vi "Score L3.vi"(9 "Combo Box":string(combo)) -> (0 "Done":bool)   [LabVIEW 2020]
uses:
  <vilib>/Rock Robotics/WPI/Utilities/WPI_GetSetVariantRefNum.vi
  Robot Global Data.vi
  <vilib>/Rock Robotics/WPI/RobotDrive/WPI_RobotDriveArcadeDrive_Standard(NoSaturation).vi
panel:
  out "Done":bool
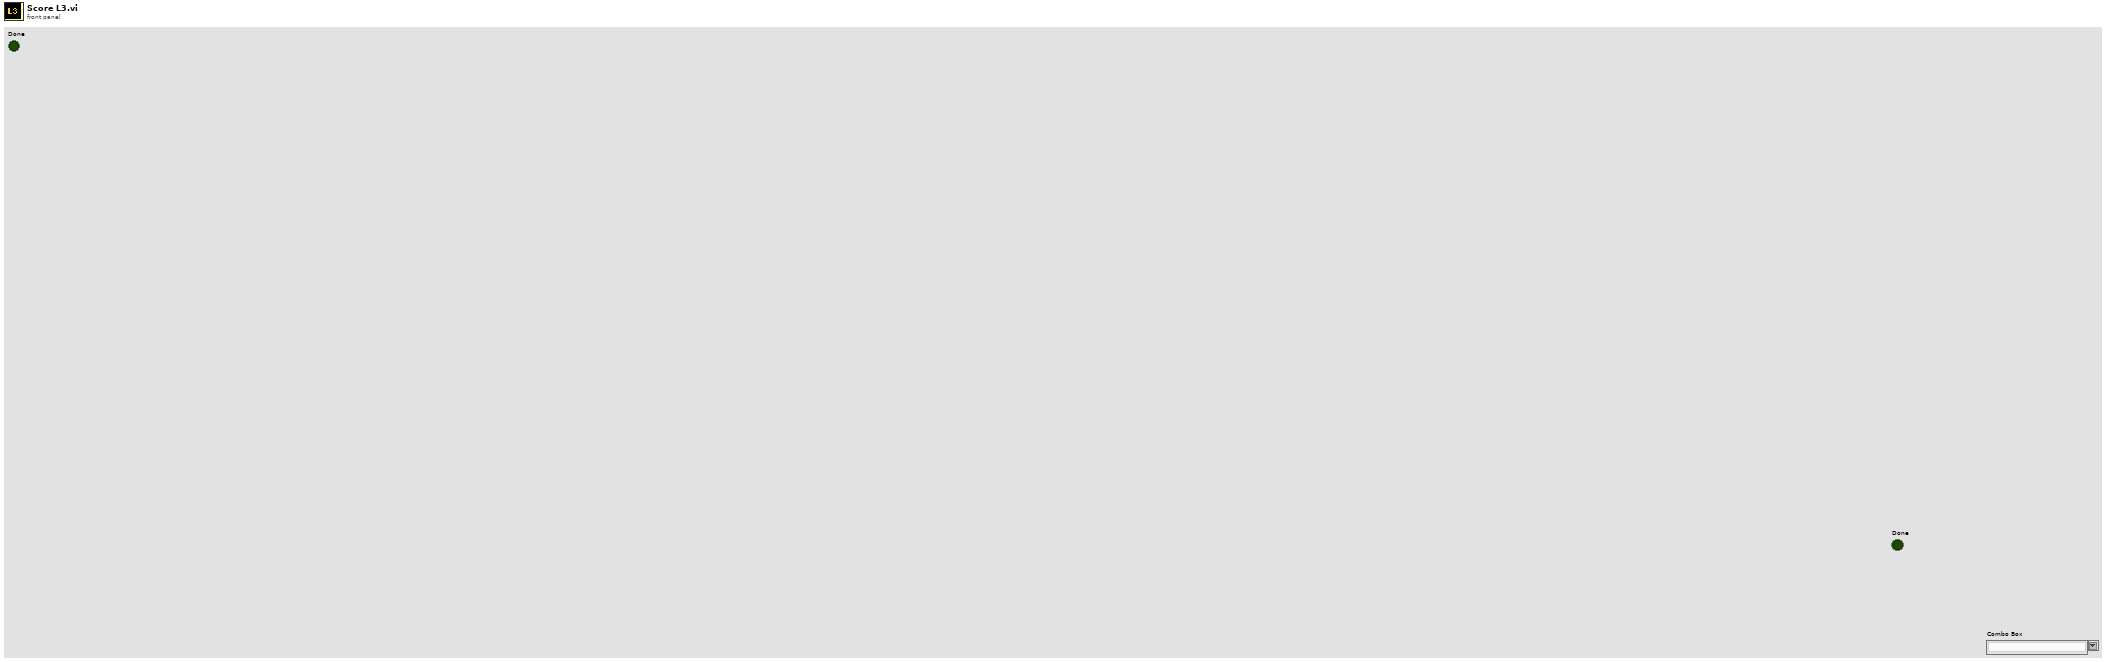
[diagram p1: front panel]
types:
  T1 = typedef "WPI_MotorControlDeviceRef.ctl" = cluster{"DeviceStatus":errorcluster, "Type":T2, "PWM":cluster{"PWM Channel":T3, "DeadBand":T4}, "CAN":cluster{"Device Number":u8, "SetOutput VI Ref":variant, "GetOutput VI Ref":variant, "Enable VI Ref":variant, "Disable VI Ref":variant, "Data":variant}, "Invert":bool, "DIO PWM":cluster{"PWM \"Enable\" Channel":T3, "DIOChannel":T5, "PWM Rate":dbl}}
  T2 = typedef "WPI_MotorControlType.ctl" = enum16{"PWM", "CAN", "DIO PWM"}
  T3 = typedef "FPGA_DIOPWMChannel.ctl" = enum8{"PWM 0", "PWM 1", "PWM 2", "PWM 3", "PWM 4", "PWM 5", "PWM 6", "PWM 7", "PWM 8", "PWM 9", "PWM MXP 0", "PWM MXP 1", "PWM MXP 2", "PWM MXP 3", "PWM MXP 4", "PWM MXP 5", "PWM MXP 6", "PWM MXP 7", "PWM MXP 8", "PWM MXP 9", "Invalid"}
  T4 = typedef "WPI_PWMDeadband.ctl" = cluster{"Name":string, "maxPositivePwm":i32, "minPositivePwm":i32, "centerPwm":i32, "maxNegativePwm":i32, "minNegativePwm":i32, "angularRange":u16}
  T5 = typedef "FPGA_DIOChannel.ctl" = enum8{"DIO 0", "DIO 1", "DIO 2", "DIO 3", "DIO 4", "DIO 5", "DIO 6", "DIO 7", "DIO 8", "DIO 9", "DIO MXP 0", "DIO MXP 1", "DIO MXP 2", "DIO MXP 3", "DIO MXP 4", "DIO MXP 5", "DIO MXP 6", "DIO MXP 7", "DIO MXP 8", "DIO MXP 9", "DIO MXP 10", "DIO MXP 11", "DIO MXP 12", "DIO MXP 13", "DIO MXP 14", "DIO MXP 15", "SPI Port CS1", "SPI Port CS2", "SPI Port CS3", "SPI Port MISO", "SPI Port MOSI", "Invalid"}
  T6 = typedef "ADIS16470 Device Reference.ctl" = cluster{"DevStatus":errorcluster, "Hardware Config":T7, "Calibration Complete":refnum<notifier>, "Status Reference":refnum<data-value>, "Data Reference":refnum<data-value>, "Sychronous Process VI":T10, "Cmd FIFO":refnum<k33>, "Source":T11, "Data FIFO":refnum<k33>, "Calibration Time (ms)":u32, "Data Reference":refnum<data-value>}
  T7 = typedef "ADIS16470 Hardware Configuration.ctl" = cluster{"SPI Clock Rate (Hz)":dbl, "IMU SPI Mode (3)":T8, "IMU Reset Pin":T5, "IMU SPI Bus":T9, "IMU Data Ready Pin":T5, "Stall Config":cluster{"Pow2BytesPerRead":u8, "StallTicks":u16, "CsToSclkTicks":u8}}
  T8 = typedef "WPI_SPIMode.ctl" = enum16{"Mode 0 (Clk Idle Low,Sample on Leading)", "Mode 1 (Clk Idle Low,Sample on Trailing)", "Mode 2 (Clk Idle High,Sample on Leading)", "Mode 3 (Clk Idle High,Sample on Trailing)"}
  T9 = typedef "spi_bus.ctl" = enum16{"SPI On-Board, CS0", "SPI On-Board, CS1", "SPI On-Board, CS2", "SPI On-Board, CS3", "SPI MXP", "Invalid"}
  T10 = typedef "ADIS16470 Process.ctl" = refnum<vi>
  T11 = typedef "FPGA_CounterEncoderSourceConvertionLVSourceType.ctl" = cluster{"DevStatus":errorcluster, "AnalogTriggerMode?":bool, "DigitalMode":cluster{"DIO Channel":T12}, "AnalogTriggerMode":cluster{"AnalogTriggerIndex":T13, "OutputType":T14}}
  T12 = typedef "FPGA_DIODigitalSourceChannel.ctl" = enum8{"DIO 0", "DIO 1", "DIO 2", "DIO 3", "DIO 4", "DIO 5", "DIO 6", "DIO 7", "DIO 8", "DIO 9", "DIO MXP 0", "DIO MXP 1", "DIO MXP 2", "DIO MXP 3", "DIO MXP 4", "DIO MXP 5", "DIO MXP 6", "DIO MXP 7", "DIO MXP 8", "DIO MXP 9", "DIO MXP 10", "DIO MXP 11", "DIO MXP 12", "DIO MXP 13", "DIO MXP 14", "DIO MXP 15", "SPI Port CS1", "SPI Port CS2", "SPI Port CS3", "SPI Port MISO", "SPI Port MOSI", "Disabled"}
  T13 = typedef "FPGA_AnalogTriggerIndex.ctl" = enum8{"Trig 0", "Trig 1", "Trig 2", "Trig 3", "Trig 4", "Trig 5", "Trig 6", "Trig 7", "Invalid"}
  T14 = typedef "FPGA_AnalogTriggerOutType.ctl" = enum16{"InWindow", "TriggerState", "Rising", "Falling"}
  T15 = typedef "WPI_RobotDriveDevRef.ctl" = cluster{"DevStatus":errorcluster, "Motors[]":T1[], "Square Inputs":bool, "Max Output":dbl}
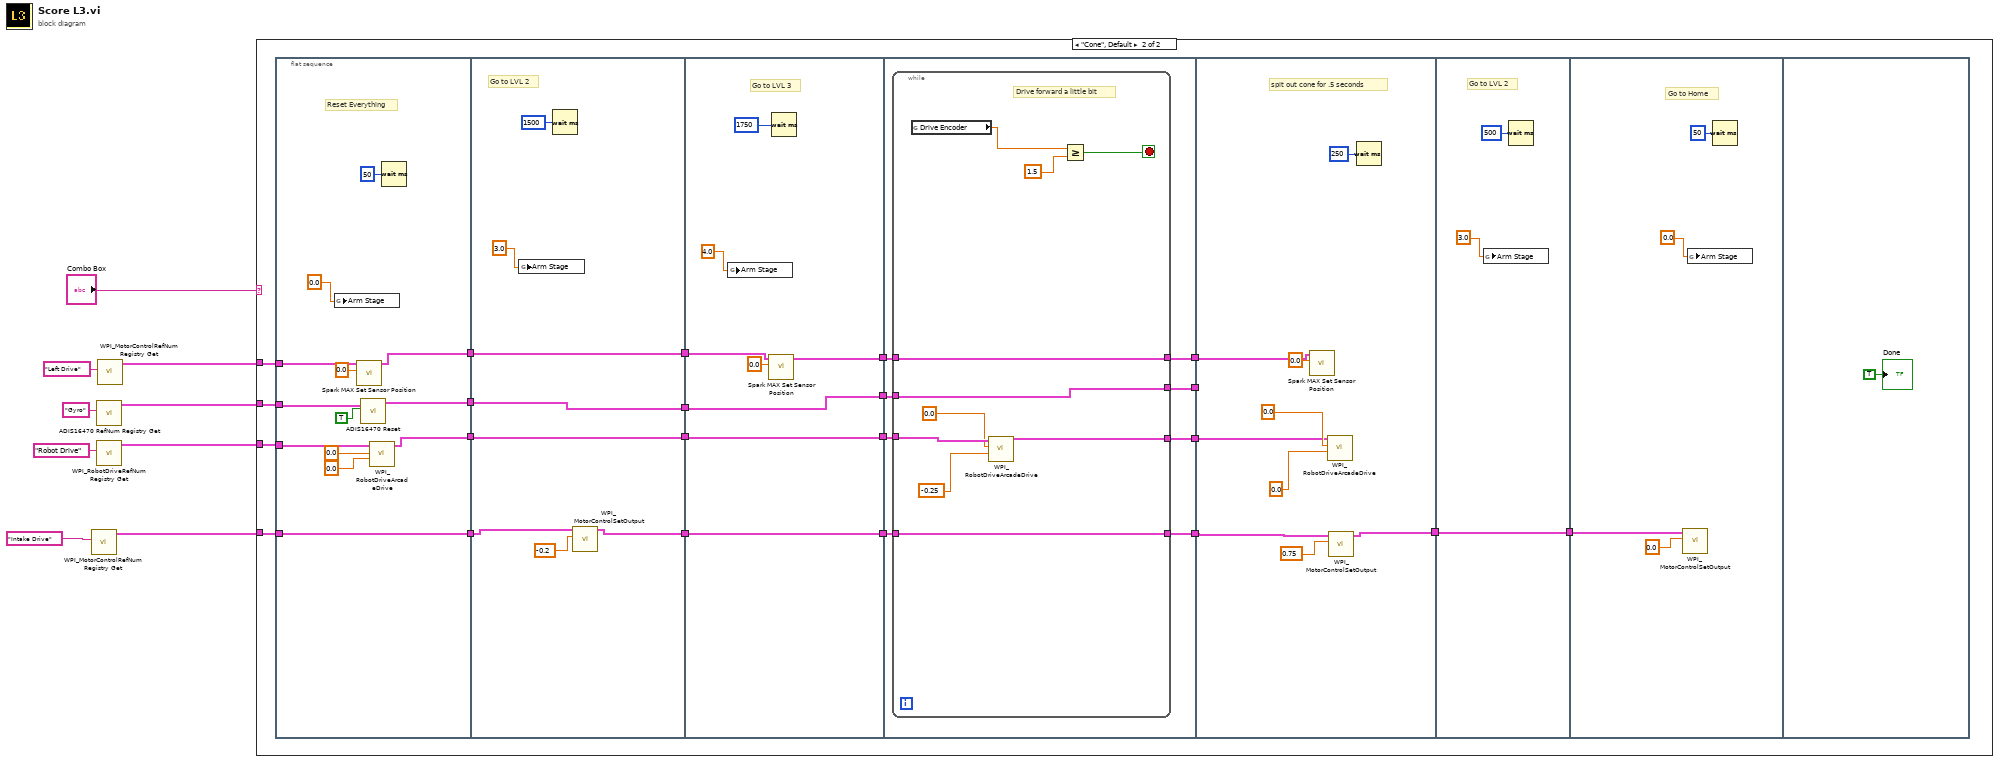
[diagram p0: block diagram]
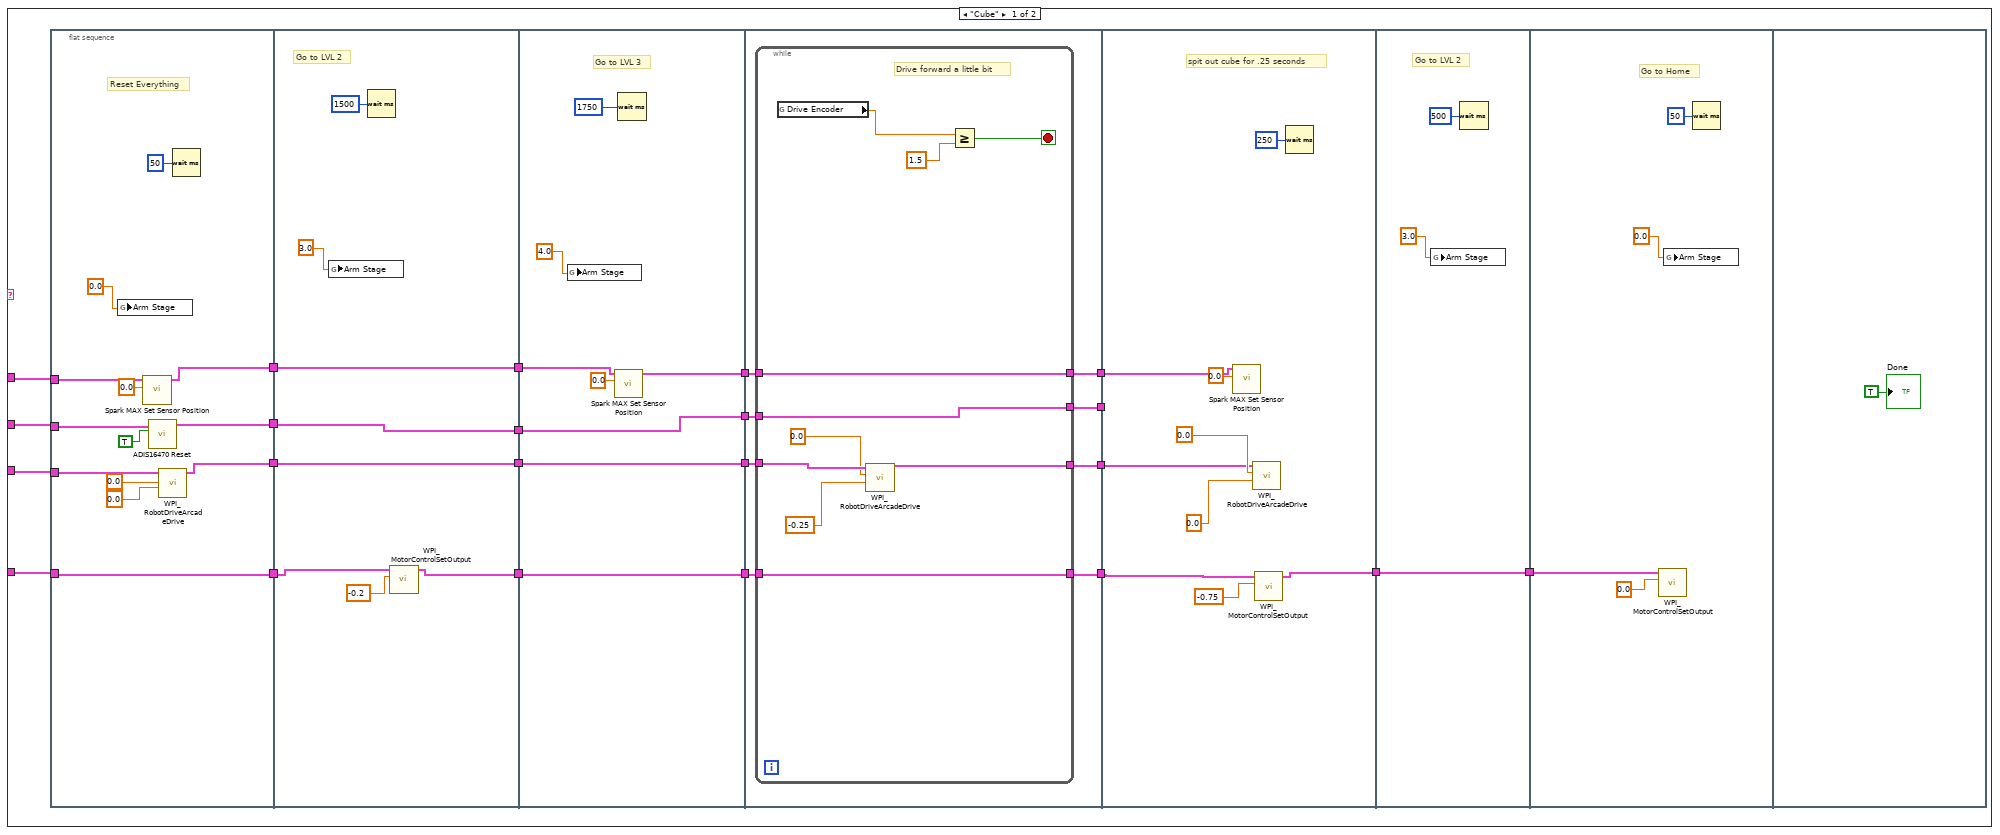
[diagram p2: hidden frame]
diagram:
  n1 = call <vilib>:"WPI_MotorControlRefNum Registry Get.vi"("refnum name"="Intake Drive") -> ("MotorControlDevRef"=w2:T1)  [unwired: 9 in, 1 out]
  n2 = call <vilib>:"ADIS16470 RefNum Registry Get.vi"("refnum name"="Gyro") -> ("ADIS16470DevRef out"=w4:T6)  [unwired: 9 in, 1 out]
  n3 = call <vilib>:"WPI_RobotDriveRefNum Registry Get.vi"("refnum name"="Robot Drive") -> ("RobotDriveDevRef"=w3:T15)  [unwired: 9 in, 1 out]
  n4 = call <vilib>:"WPI_MotorControlRefNum Registry Get.vi"("refnum name"="Left Drive") -> ("MotorControlDevRef"=w5:T1)  [unwired: 9 in, 1 out]
  n5 = case shown="\"Cone\", Default" "Combo Box" {
    tunnel: w5 -> [w13 w99]
    tunnel: w4 -> [w12 w98]
    tunnel: w3 -> [w11 w97]
    tunnel: w2 -> [w10 w96]
    frame "Cube" {
      n6 = flat-sequence {
        tunnel: w11 -> [w44]
        tunnel: w13 -> [w41]
        tunnel: w12 -> [w39]
        tunnel: [w35] -> w31
        tunnel: [w34] -> w30
        tunnel: w10 -> [w34]
        tunnel: [w33] -> w29
        tunnel: [w32] -> w28
        tunnel: [w50] -> w27
        tunnel: w31 -> [w50]
        tunnel: w30 -> [w46]
        tunnel: [w45] -> w26
        tunnel: [w49] -> w25
        tunnel: w29 -> [w49]
        tunnel: [w48] -> w24
        tunnel: w28 -> [w48]
        tunnel: [w58] -> w23
        tunnel: w27 -> [w58]
        tunnel: [w53] -> w22
        tunnel: w26 -> [w53]
        tunnel: w25 -> [w56]
        tunnel: [w55] -> w21
        tunnel: [w54] -> w20
        tunnel: w24 -> [w54]
        tunnel: w23 -> [w68]
        tunnel: w22 -> [w67]
        tunnel: [w66] -> w19
        tunnel: [w65] -> w18
        tunnel: [w64] -> w17
        tunnel: w21 -> [w63]
        tunnel: [w62] -> w16
        tunnel: w20 -> [w61]
        tunnel: w19 -> [w84]
        tunnel: w18 -> [w83]
        tunnel: w17 -> [w80]
        tunnel: w16 -> [_]
        tunnel: [w79] -> w15
        tunnel: [w88] -> w14
        tunnel: w15 -> [w88]
        tunnel: w14 -> [w92]
        frame #0 {
          # "Reset Everything"
          n7 = global write "Robot Global Data.vi" "Arm Stage"(0.0 ("Arm Stage")) -> ()
          n8 = call <vilib>:"Spark MAX Set Sensor Position.vi"("Position"=0.0, "MotorControlDeviceRef"=w41) -> ("MotorControlDeviceRef"=w33:T1)  [unwired: 8 in, 1 out]
          n9 = call <vilib>:"ADIS16470 Reset.vi"("Reset? (T)"=TRUE, "ADIS16470DevRef"=w39) -> ("ADIS16470DevRef"=w32:T6)  [unwired: 8 in, 1 out]
          n10 = call-poly <vilib>:"WPI_RobotDriveArcadeDrive.vi"("Y axis value"=0.0, "X axis value"=0.0, "RobotDriveDevRef"=w44) -> ("RobotDriveDevRef"=w35:T15)  [unwired: 6 in, 2 out]
          n11 = Wait (ms)(milliseconds to wait=u32 50) -> ()  [unwired: 1 out]
        }
        frame #1 {
          # "Go to LVL 2"
          n12 = global write "Robot Global Data.vi" "Arm Stage"(3.0 ("Arm Stage")) -> ()
          n13 = Wait (ms)(milliseconds to wait=u32 1500) -> ()  [unwired: 1 out]
          n14 = call <vilib>:"WPI_MotorControlSetOutput.vi"("Output"=-0.2, "MotorControlDevRef"=w46) -> ("MotorControlDevRef"=w45:T1)  [unwired: 7 in, 2 out]
        }
        frame #2 {
          # "Go to LVL 3"
          n15 = global write "Robot Global Data.vi" "Arm Stage"(4.0 ("Arm Stage")) -> ()
          n16 = call <vilib>:"Spark MAX Set Sensor Position.vi"("Position"=0.0, "MotorControlDeviceRef"=w56) -> ("MotorControlDeviceRef"=w55:T1)  [unwired: 8 in, 1 out]
          n17 = Wait (ms)(milliseconds to wait=u32 1750) -> ()  [unwired: 1 out]
        }
        frame #3 {
          n18 = while {
            tunnel: w68 -> [w78]
            tunnel: w67 -> [w72]
            tunnel: [w72] -> w66
            tunnel: [w71] -> w65
            tunnel: [w70] -> w64
            tunnel: w63 -> [w70]
            tunnel: [w69] -> w62
            tunnel: w61 -> [w69]
            stop <- w73 stop-if-true
            # "Drive forward a little bit"
            n19 = global read "Robot Global Data.vi" "Drive Encoder"() -> (w75:dbl)
            n20 = call-poly <vilib>:"WPI_RobotDriveArcadeDrive.vi"("Y axis value"=-0.25, "X axis value"=0.0, "RobotDriveDevRef"=w78) -> ("RobotDriveDevRef"=w71:T15)  [unwired: 6 in, 2 out]
            n21 = Greater Or Equal?(x=w75, y=1.5) -> (x >= y?=w73:bool)
          }
        }
        frame #4 {
          # "spit out cube for .25 seconds"
          n22 = call <vilib>:"Spark MAX Set Sensor Position.vi"("Position"=0.0, "MotorControlDeviceRef"=w80) -> ()  [unwired: 8 in, 2 out]
          n23 = call-poly <vilib>:"WPI_RobotDriveArcadeDrive.vi"("Y axis value"=0.0, "X axis value"=0.0, "RobotDriveDevRef"=w83) -> ()  [unwired: 6 in, 3 out]
          n24 = call <vilib>:"WPI_MotorControlSetOutput.vi"("Output"=-0.75, "MotorControlDevRef"=w84) -> ("MotorControlDevRef"=w79:T1)  [unwired: 7 in, 2 out]
          n25 = Wait (ms)(milliseconds to wait=u32 250) -> ()  [unwired: 1 out]
        }
        frame #5 {
          # "Go to LVL 2"
          n26 = global write "Robot Global Data.vi" "Arm Stage"(3.0 ("Arm Stage")) -> ()
          n27 = Wait (ms)(milliseconds to wait=u32 500) -> ()  [unwired: 1 out]
        }
        frame #6 {
          # "Go to Home"
          n28 = call <vilib>:"WPI_MotorControlSetOutput.vi"("Output"=0.0, "MotorControlDevRef"=w92) -> ()  [unwired: 7 in, 3 out]
          n29 = global write "Robot Global Data.vi" "Arm Stage"(0.0 ("Arm Stage")) -> ()
          n30 = Wait (ms)(milliseconds to wait=u32 50) -> ()  [unwired: 1 out]
        }
        frame #7 {
          "Done" <- TRUE ("Done")
        }
      }
    }
    frame "Cone", Default {
      n31 = flat-sequence {
        tunnel: w97 -> [w130]
        tunnel: w99 -> [w127]
        tunnel: w98 -> [w125]
        tunnel: [w121] -> w117
        tunnel: [w120] -> w116
        tunnel: w96 -> [w120]
        tunnel: [w119] -> w115
        tunnel: [w118] -> w114
        tunnel: [w136] -> w113
        tunnel: w117 -> [w136]
        tunnel: w116 -> [w132]
        tunnel: [w131] -> w112
        tunnel: [w135] -> w111
        tunnel: w115 -> [w135]
        tunnel: [w134] -> w110
        tunnel: w114 -> [w134]
        tunnel: [w144] -> w109
        tunnel: w113 -> [w144]
        tunnel: [w139] -> w108
        tunnel: w112 -> [w139]
        tunnel: w111 -> [w142]
        tunnel: [w141] -> w107
        tunnel: [w140] -> w106
        tunnel: w110 -> [w140]
        tunnel: w109 -> [w154]
        tunnel: w108 -> [w153]
        tunnel: [w152] -> w105
        tunnel: [w151] -> w104
        tunnel: [w150] -> w103
        tunnel: w107 -> [w149]
        tunnel: [w148] -> w102
        tunnel: w106 -> [w147]
        tunnel: w105 -> [w170]
        tunnel: w104 -> [w169]
        tunnel: w103 -> [w166]
        tunnel: w102 -> [_]
        tunnel: [w165] -> w101
        tunnel: [w174] -> w100
        tunnel: w101 -> [w174]
        tunnel: w100 -> [w178]
        frame #0 {
          # "Reset Everything"
          n32 = global write "Robot Global Data.vi" "Arm Stage"(0.0 ("Arm Stage")) -> ()
          n33 = call <vilib>:"Spark MAX Set Sensor Position.vi"("Position"=0.0, "MotorControlDeviceRef"=w127) -> ("MotorControlDeviceRef"=w119:T1)  [unwired: 8 in, 1 out]
          n34 = call <vilib>:"ADIS16470 Reset.vi"("Reset? (T)"=TRUE, "ADIS16470DevRef"=w125) -> ("ADIS16470DevRef"=w118:T6)  [unwired: 8 in, 1 out]
          n35 = call-poly <vilib>:"WPI_RobotDriveArcadeDrive.vi"("Y axis value"=0.0, "X axis value"=0.0, "RobotDriveDevRef"=w130) -> ("RobotDriveDevRef"=w121:T15)  [unwired: 6 in, 2 out]
          n36 = Wait (ms)(milliseconds to wait=u32 50) -> ()  [unwired: 1 out]
        }
        frame #1 {
          # "Go to LVL 2"
          n37 = global write "Robot Global Data.vi" "Arm Stage"(3.0 ("Arm Stage")) -> ()
          n38 = Wait (ms)(milliseconds to wait=u32 1500) -> ()  [unwired: 1 out]
          n39 = call <vilib>:"WPI_MotorControlSetOutput.vi"("Output"=-0.2, "MotorControlDevRef"=w132) -> ("MotorControlDevRef"=w131:T1)  [unwired: 7 in, 2 out]
        }
        frame #2 {
          # "Go to LVL 3"
          n40 = global write "Robot Global Data.vi" "Arm Stage"(4.0 ("Arm Stage")) -> ()
          n41 = call <vilib>:"Spark MAX Set Sensor Position.vi"("Position"=0.0, "MotorControlDeviceRef"=w142) -> ("MotorControlDeviceRef"=w141:T1)  [unwired: 8 in, 1 out]
          n42 = Wait (ms)(milliseconds to wait=u32 1750) -> ()  [unwired: 1 out]
        }
        frame #3 {
          n43 = while {
            tunnel: w154 -> [w164]
            tunnel: w153 -> [w158]
            tunnel: [w158] -> w152
            tunnel: [w157] -> w151
            tunnel: [w156] -> w150
            tunnel: w149 -> [w156]
            tunnel: [w155] -> w148
            tunnel: w147 -> [w155]
            stop <- w159 stop-if-true
            # "Drive forward a little bit"
            n44 = global read "Robot Global Data.vi" "Drive Encoder"() -> (w161:dbl)
            n45 = call-poly <vilib>:"WPI_RobotDriveArcadeDrive.vi"("Y axis value"=-0.25, "X axis value"=0.0, "RobotDriveDevRef"=w164) -> ("RobotDriveDevRef"=w157:T15)  [unwired: 6 in, 2 out]
            n46 = Greater Or Equal?(x=w161, y=1.5) -> (x >= y?=w159:bool)
          }
        }
        frame #4 {
          # "spit out cone for .5 seconds"
          n47 = call <vilib>:"Spark MAX Set Sensor Position.vi"("Position"=0.0, "MotorControlDeviceRef"=w166) -> ()  [unwired: 8 in, 2 out]
          n48 = call-poly <vilib>:"WPI_RobotDriveArcadeDrive.vi"("Y axis value"=0.0, "X axis value"=0.0, "RobotDriveDevRef"=w169) -> ()  [unwired: 6 in, 3 out]
          n49 = call <vilib>:"WPI_MotorControlSetOutput.vi"("Output"=0.75, "MotorControlDevRef"=w170) -> ("MotorControlDevRef"=w165:T1)  [unwired: 7 in, 2 out]
          n50 = Wait (ms)(milliseconds to wait=u32 250) -> ()  [unwired: 1 out]
        }
        frame #5 {
          # "Go to LVL 2"
          n51 = global write "Robot Global Data.vi" "Arm Stage"(3.0 ("Arm Stage")) -> ()
          n52 = Wait (ms)(milliseconds to wait=u32 500) -> ()  [unwired: 1 out]
        }
        frame #6 {
          # "Go to Home"
          n53 = call <vilib>:"WPI_MotorControlSetOutput.vi"("Output"=0.0, "MotorControlDevRef"=w178) -> ()  [unwired: 7 in, 3 out]
          n54 = global write "Robot Global Data.vi" "Arm Stage"(0.0 ("Arm Stage")) -> ()
          n55 = Wait (ms)(milliseconds to wait=u32 50) -> ()  [unwired: 1 out]
        }
        frame #7 {
          "Done" <- TRUE ("Done")
        }
      }
    }
  }
